vi "MicroblazeExample_Download.vi"() -> ()   [LabVIEW 2015]
uses:
  UART_1_0_0/Settings.ctl
  UART_1_0_0/Parity.ctl
  UART_1_0_0/StopBits.ctl
  <vilib>/Platform/TimedLoop/XDataNode/timing_clust.ctl
  <vilib>/Platform/TimedLoop/XDataNode/nitl_modes.ctl
  <vilib>/Platform/TimedLoop/XDataNode/wakeup.ctl
  <vilib>/rvi/Emulation/niFpgaSctlEmulationGetInTimedLoop.vi
  <vilib>/rvi/Emulation/niFpgaEmulationReportErrorSimple.vi
  <vilib>/rvi/Emulation/niFpgaGetClockAttributes.vi
  <vilib>/rvi/Emulation/niFpgaCriticalErrorInLSC.vi
  <vilib>/rvi/eio/common/nirviEmuTemplateMethod_errors.vi
  <vilib>/rvi/interface/RandomDataEmulation/niFpgaRandomDataHandleErrors.vi
  <vilib>/Platform/TimedLoop/XDataNode/XDataNode.xnode
  <vilib>/eio/EIONode/EIONode.xnode
  <vilib>/rvi/DataTransferAndStorage/Container/XNode/niFpgaContainer.xnode
  <vilib>/rvi/interface/RandomDataEmulation/nirviRandomDataFpgaReadWriteTemplate.vi
  <vilib>/Platform/TimedLoop/XDataNode/XDNodeRunTimeDep.lvlib
  UART_1_0_0/UART_Firmware.lvlib
panel:
  in  "ub1\\BRAM_PORTB_en":bool
  in  "ub1\\BRAM_PORTB_rst":bool
  in  "ub1\\BRAM_PORTB_we":fxp<+,4,4>=15.0 format="%.0b"
  in  "ub1\\reset_rtl":bool
  in  "A":u32
  in  "B":u32
  out "C":u32
  in  "ub1\\uart_rtl_rxd":bool
  in  "Settings":T1={"Baud (ticks)"=868, "CharacterSize"=8, "Parity"=enum."None", "Stop Bits"=enum."1.0", "Spacing (ticks)"=0}
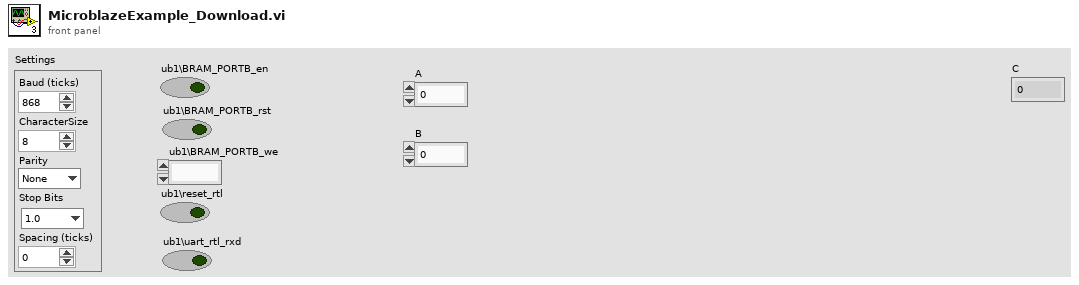
[diagram p1: front panel]
types:
  T1 = typedef "UART_Firmware.lvlib/Settings.ctl" = cluster{"Baud (ticks)":u32, "CharacterSize":u8, "Parity":T2, "Stop Bits":T3, "Spacing (ticks)":u32}
  T2 = typedef "UART_Firmware.lvlib/Parity.ctl" = enum8{"None", "Even", "Odd"}
  T3 = typedef "UART_Firmware.lvlib/StopBits.ctl" = enum8{"1.0", "1.5", "2.0"}
  T4 = typedef "XDNodeRunTimeDep.lvlib/timing_clust.ctl" = cluster{"Expected End [f-1]":u64, "Actual End [f-1]":u64, "Finished Late? [f-1]":bool, "Expected End [i-1]":u64, "Actual End [i-1]":u64, "Finished Late? [i-1]":bool, "Expected Start [i]":u64, "Actual Start [i]":u64, "Expected Start [f]":u64, "Actual Start [f]":u64, "Source Name":string, "Structure Name":string, "Period":i64, "Deadline":i64, "Offset":i64, "Start":i64, "Priority":i32, "Timeout":i32, "Mode":T5, "Wakeup Reason":T6, "Error":errorcluster, "Source Type":string, "Secondary Source Type":string, "Global End Time":u64, "Global Start Time":u64, "Frame Duration":u64, "Iteration Duration":u64, "Assigned CPU":i32, "I/O Scan Engine Mode":u32}
  T5 = typedef "XDNodeRunTimeDep.lvlib/nitl_modes.ctl" = enum32{"No Change", "Process missed periods, maintain original phase", "Discard missed periods, maintain original phase", "Process missed periods, ignore original phase", "Discard missed periods, ignore original phase"}
  T6 = typedef "XDNodeRunTimeDep.lvlib/wakeup.ctl" = enum32{"Normal", "Aborted", "Asynchronous wakeup", "Timing source error", "Timed loop error", "Timeout"}
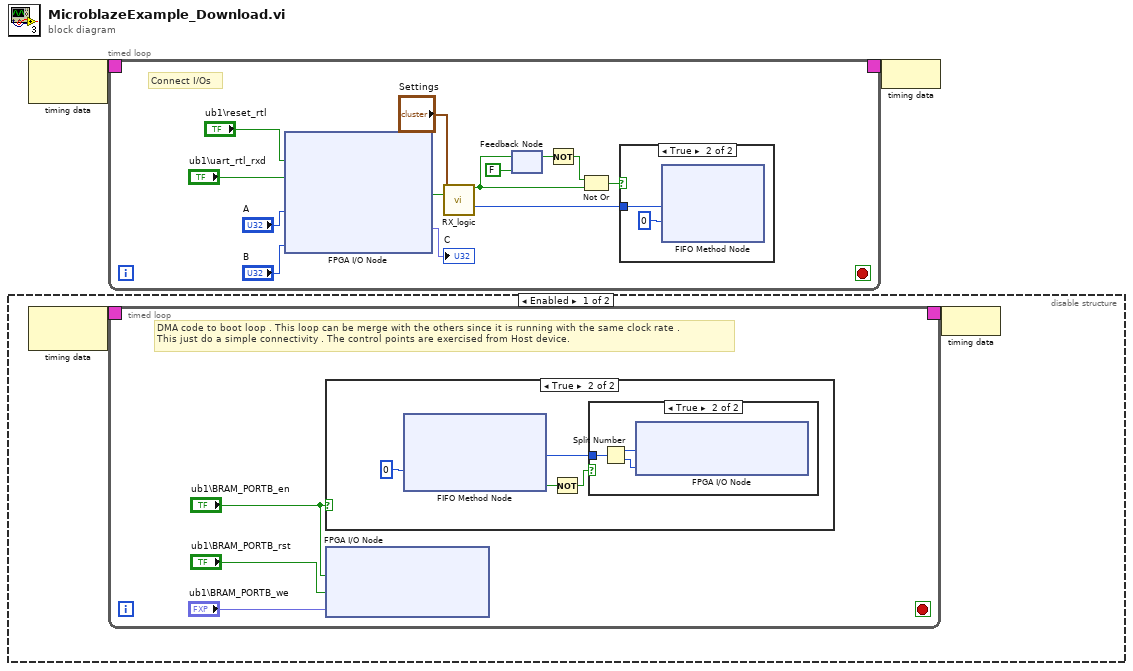
[diagram p0: block diagram]
diagram:
  n1 = disable-structure shown="Enabled" {
    frame Enabled {
      n2 = node-c288() -> (w4:T4)  [unwired: 1 in]
      n3 = timed-loop {
        timing: w4 -> [_]
        timing-out: [_] -> w3
        stop <- _ stop-if-true
        # "DMA code to boot loop . This loop can be merge with the others since it is running with the same clock rate . \nThis just do a simple connectivity . The control points are exercised from Host device."
        n4 = case shown="True" "ub1\\BRAM_PORTB_en" {
          frame False {
          }
          frame True {
            n5 = xnode ("FIFO Method Node")("Timeout"=0) -> ("Element"=w10:i16, "Timed Out?"=w9:bool)  [unwired: 1 in, 1 out]
            n6 = Not(x=w9) -> (.not. x?=w8:bool)
            n7 = case shown="True" w8 {
              tunnel: w10 -> [_ w14]
              frame False {
              }
              frame True {
                n8 = Split Number(x=w14) -> (hi(x)=w13:u8, lo(x)=w12:u8)
                n9 = xnode "FPGA I/O Node"("ub1\\BRAM_PORTB_addr"=w13, "ub1\\BRAM_PORTB_din"=w12) -> ()  [unwired: 2 in, 2 out]
              }
            }
          }
        }
        n10 = xnode "FPGA I/O Node"("ub1\\BRAM_PORTB_en"="ub1\\BRAM_PORTB_en", "ub1\\BRAM_PORTB_rst"="ub1\\BRAM_PORTB_rst", "ub1\\BRAM_PORTB_we"="ub1\\BRAM_PORTB_we") -> ()  [unwired: 3 in, 3 out]
      }
      n11 = node-c288(w3) -> ()
    }
    frame Disabled {
    }
  }
  n12 = node-c288() -> (w2:T4)  [unwired: 1 in]
  n13 = timed-loop {
    timing: w2 -> [_]
    timing-out: [_] -> w1
    stop <- _ stop-if-true
    # "Connect I/Os"
    n14 = xnode "FPGA I/O Node"("ub1\\reset_rtl"="ub1\\reset_rtl", "ub1\\uart_rtl_rxd"="ub1\\uart_rtl_rxd", "ub1\\gpio_rtl_0_tri_i"="A", "ub1\\gpio_rtl_tri_i"="B") -> ("ub1\\uart_rtl_txd"=w27:bool, "ub1\\gpio_rtl_1_tri_o"=→"C":fxp<+,32,32>)  [unwired: 6 in, 6 out]
    n15 = call "RX_logic.vi"("Settings"="Settings", "Rx"=w27) -> ("Busy"=w23:bool, "Rx_data"=w21:u16)  [unwired: 10 in, 2 out]
    n16 = feedback-in #1(w23) -> ()
    n17 = feedback #1(FALSE ("Busy")) -> (w25:bool)
    n18 = Not(x=w25) -> (.not. x?=w22:bool)
    n19 = Not Or(1:w23, 2:w22) -> (0:w24:bool)
    n20 = case shown="True" w24 {
      tunnel: w21 -> [_ w32]
      frame False {
      }
      frame True {
        n21 = xnode ("FIFO Method Node")("Element"=w32, "Timeout"=0) -> ()  [unwired: 1 in, 2 out]
      }
    }
  }
  n22 = node-c288(w1) -> ()
